vi "HistoryAverages.vi"(11 "History Data":T1(array[cluster])) -> (3 "Averages":dbl[](array[numeric]))   [LabVIEW 2024]
uses:
  <vilib>/Analysis/baseanly.llb/Mean (DBL).vi
  <vilib>/Analysis/NI_AALBase.lvlib
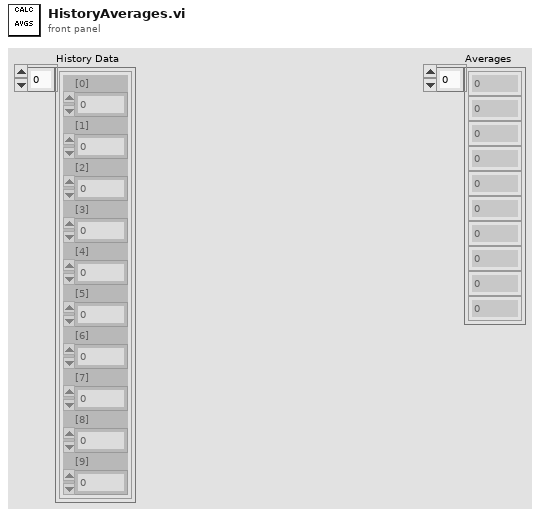
[diagram p1: front panel]
types:
  T1 = cluster{"[0]":dbl, "[1]":dbl, "[2]":dbl, "[3]":dbl, "[4]":dbl, "[5]":dbl, "[6]":dbl, "[7]":dbl, "[8]":dbl, "[9]":dbl}[]
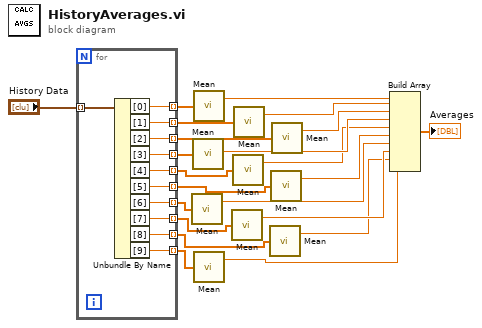
[diagram p0: block diagram]
diagram:
  n1 = for {
    tunnel: "History Data" -> [w33] mode=indexing
    tunnel: [w32] -> w22 mode=indexing
    tunnel: [w31] -> w21 mode=indexing
    tunnel: [w30] -> w20 mode=indexing
    tunnel: [w29] -> w19 mode=indexing
    tunnel: [w28] -> w18 mode=indexing
    tunnel: [w27] -> w17 mode=indexing
    tunnel: [w26] -> w16 mode=indexing
    tunnel: [w25] -> w15 mode=indexing
    tunnel: [w24] -> w14 mode=indexing
    tunnel: [w23] -> w13 mode=indexing
    n2 = Unbundle By Name(w33) -> ("[0]"=w32:dbl, "[1]"=w31:dbl, "[2]"=w30:dbl, "[3]"=w29:dbl, "[4]"=w28:dbl, "[5]"=w27:dbl, "[6]"=w26:dbl, "[7]"=w25:dbl, "[8]"=w24:dbl, "[9]"=w23:dbl)
  }
  n3 = call-poly <vilib>:"Mean.vi"("X"=w16) -> ("mean"=w6:dbl)  [unwired: 1 out]
  n4 = call-poly <vilib>:"Mean.vi"("X"=w19) -> ("mean"=w9:dbl)  [unwired: 1 out]
  n5 = call-poly <vilib>:"Mean.vi"("X"=w22) -> ("mean"=w12:dbl)  [unwired: 1 out]
  n6 = call-poly <vilib>:"Mean.vi"("X"=w13) -> ("mean"=w3:dbl)  [unwired: 1 out]
  n7 = call-poly <vilib>:"Mean.vi"("X"=w15) -> ("mean"=w5:dbl)  [unwired: 1 out]
  n8 = call-poly <vilib>:"Mean.vi"("X"=w18) -> ("mean"=w8:dbl)  [unwired: 1 out]
  n9 = call-poly <vilib>:"Mean.vi"("X"=w21) -> ("mean"=w11:dbl)  [unwired: 1 out]
  n10 = call-poly <vilib>:"Mean.vi"("X"=w14) -> ("mean"=w4:dbl)  [unwired: 1 out]
  n11 = call-poly <vilib>:"Mean.vi"("X"=w17) -> ("mean"=w7:dbl)  [unwired: 1 out]
  n12 = call-poly <vilib>:"Mean.vi"("X"=w20) -> ("mean"=w10:dbl)  [unwired: 1 out]
  n13 = Build Array(w12, w11, w10, w9, w8, w7, w6, w5, w4, w3) -> (→"Averages":dbl[])
